vi "PCO_GetCmosLineExposureDelay.vi"(8 "error in (no error)":errorcluster {"code" format="%x"}, 11 "ph":u64) -> (0 "error out":errorcluster {"code" format="%x"}, 1 "dwExposureLines":u32, 2 "ErrorMessage":i32 format="%x", 3 "ph out":u64, 5 "dwDelayLines":u32)   [LabVIEW 2020, in "SDK.lvlib" / "SpecialCommandsEdge.lvlib"]
doc: "<b>Description:</b>\nThis function returns the current setting of the exposure and delay line settings for the Lightsheet scanning mode. It is only available when Lightsheet scanning mode has been successfully enabled by PCO_SetCmosLineTiming.\n\n<b>Supported camera type:</b>\npco.edge with Camera Link interface\n\n<b>Descriptor dependency:</b>\nNone"
uses:
  SpecialCommandsEdge.lvlib
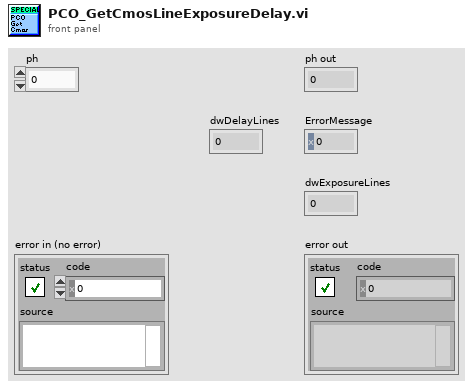
[diagram p1: front panel]
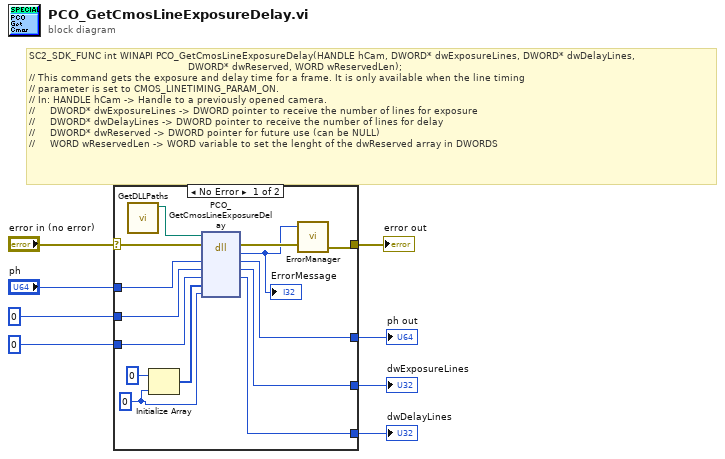
[diagram p0: block diagram]
diagram:
  # "SC2_SDK_FUNC int WINAPI PCO_GetCmosLineExposureDelay(HANDLE hCam, DWORD* dwExposureLines, DWORD* dwDelayLines,\n                                                     DWORD* dwReserved, WORD wReservedLen);\n// This command gets the exposure and delay time for a frame. It is only available when the line timing \n// parameter is set to CMOS_LINETIMING_PARAM_ON.\n// In: HANDLE hCam -> Handle to a previously opened camera.\n//     DWORD* dwExposureLines -> DWORD pointer to receive the number of lines for exposure\n//     DWORD* dwDelayLines -> DWORD pointer to receive the number of lines for delay\n//     DWORD* dwReserved -> DWORD pointer for future use (can be NULL)\n//     WORD wReservedLen -> WORD variable to set the lenght of the dwReserved array in DWORDS"
  n1 = case shown="No Error" "error in (no error)" {
    selector: "error in (no error)" -> [w13 w26]
    tunnel: "ph" -> [w22 w25]
    tunnel: [w21 w25] -> w7
    tunnel: u32 0 ("dwExposureLines") -> [w20 w24]
    tunnel: [w19 w24] -> w5
    tunnel: u32 0 ("dwDelayLines") -> [w18 w23]
    tunnel: [w17 w23] -> w3
    tunnel: [w11 w26] -> w2
    frame No Error {
      w15 = u16 0 ("dimension size")
      n2 = call "GetDLLPaths.vi"() -> ("SC2_Cam_Path"=w9:path)  [unwired: 9 in, 2 out]
      n3 = Initialize Array(u32 0, w15) -> (w14:u32[])
      n4 = dll-call lib="?" fn="PCO_GetCmosLineExposureDelay"(path in=w9, error in=w13, "ph"=w22, "dwExposureLines"=w20, "dwDelayLines"=w18, "dwReserved"=w14, "wReservedLen"=w15) -> (error out=w12:errorcluster, "return type"=w10:i32, "ph"=w21:u64, "dwExposureLines"=w19:u32, "dwDelayLines"=w17:u32)  [unwired: 3 in, 1 out]
      "ErrorMessage" <- w10
      n5 = call "ErrorManager.vi"("error in (no error)"=w12, "error code"=w10) -> ("error out"=w11:errorcluster)  [unwired: 3 in]
    }
    frame Error {
    }
  }
  "ph out" <- w7
  "dwExposureLines" <- w5
  "dwDelayLines" <- w3
  "error out" <- w2
